vi "Determine Clicked Array Element Index - Cancel Error Code 1320.vi"(7 "error in":errorcluster) -> (8 "error out":errorcluster)   [LabVIEW 2016]
doc: "Determine Clicked Array Element Index - Cancel Error Code 1320.vi\n\nDescription:\nThis VI determines determines if error code 1320 has occured, and if so, cancels the error.\n\nInputs:\nerror in - Standard error cluster.\n\nOutputs:\nerror out - standard error cluster.\n\nDeveloped By:\nMark.ridgley\nMark.Ridgley_LabVIEW.Developer@comcast.net"
uses:
  <vilib>/Utility/error.llb/DialogType.ctl
panel:
  # "Error 1320 indicates that In run mode, LabVIEW cannot get or set a property for a control part that has not been created. Since arrays drop with the caption undefined, we need to cancel this error code in case the user has not defined a caption."
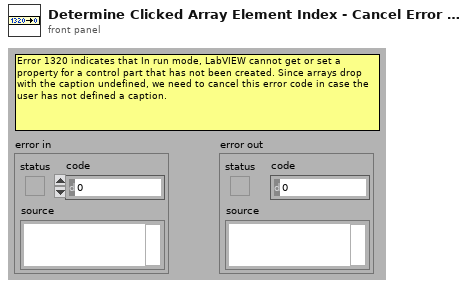
[diagram p1: front panel]
types:
  T1 = typedef "DialogType.ctl" = u16
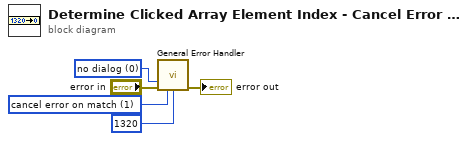
[diagram p0: block diagram]
diagram:
  w5 = T1 0 items=["no dialog", "OK message", "continue or stop message", "OK message + warnings", "continue/stop + warnings"] ("type of dialog (OK msg:1)")
  w4 = 1 items=["no exception", "cancel error on match", "set error on match"] ("[exception action] (none:0)")
  n1 = call <vilib>:"General Error Handler.vi"("type of dialog (OK msg:1)"=w5, "error in (no error)"="error in", "[exception action] (none:0)"=w4, "[exception code]"=1320) -> ("error out"=→"error out":errorcluster)  [unwired: 7 in, 4 out]
